vi "OA Delete Mode.vi"(10 "uiModeNameLen":u32, 11 "pcModeName":string) -> (3 "function return":u32)   [LabVIEW 2018, in "AndorSDK.lvlib"]
doc: "EXPNETTYPE unsigned int WINAPI OA_DeleteMode(const char * const pcModeName, unsigned int uiModeNameLen);"
uses:
  AndorSDK.lvlib
  ATMCD32D.dll
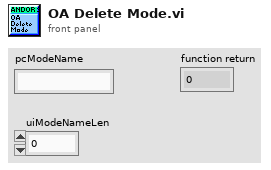
[diagram p1: front panel]
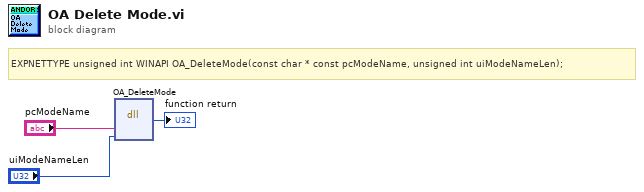
[diagram p0: block diagram]
diagram:
  # "EXPNETTYPE unsigned int WINAPI OA_DeleteMode(const char * const pcModeName, unsigned int uiModeNameLen);"
  n1 = dll-call lib="PTH2babs E\nPersönliches02 - Arbeit03-HiwijobsLabviewCodelibANDOR\tAndor SDK\nATMCD32D.*" fn="OA_DeleteMode"("pcModeName"="pcModeName", "uiModeNameLen"="uiModeNameLen") -> (→"function return":u32)  [unwired: 5 in, 2 out]
